vi "standupRoutine.vi"() -> ()   [LabVIEW 2013]
uses:
  <vilib>/Simulation/Implementation/XNodeFramework/SimXNode/SimX.xnode
  LinearControl.vi
  <vilib>/Simulation/Implementation/Shared/SIMSCR Execution Mode.ctl
  <vilib>/Simulation/Scripting/Companion Diagram/SimConfigNode/_simSolvers.ctl
  <vilib>/Simulation/Scripting/Companion Diagram/SimConfigNode/SimParams.ctl
  <vilib>/Simulation/Scripting/Companion Diagram/SimConfigNode/SimDog.xnode
panel:
  out "Dynamic Data Type":dynamicdata(graph)
  in  "SP_theta_e":dbl step=0.0001 format="%_6f"
  out "theta":dbl
  out "pos":dbl format="%.2f"
  out "Controller?":bool
  in  "state feedbak gain":dbl[](array[numeric])=[0.0, 0.0, 400.0, 0.0] step=1e-05 format="%_6f"
  in  "setpoint":dbl format="%_6g"
  in  "stop_swing":bool
  in  "stop_controller":bool
  in  "reset_theta":bool
  in  "reset_pos":bool
  in  "Start":bool
  in  "enable_swing":bool
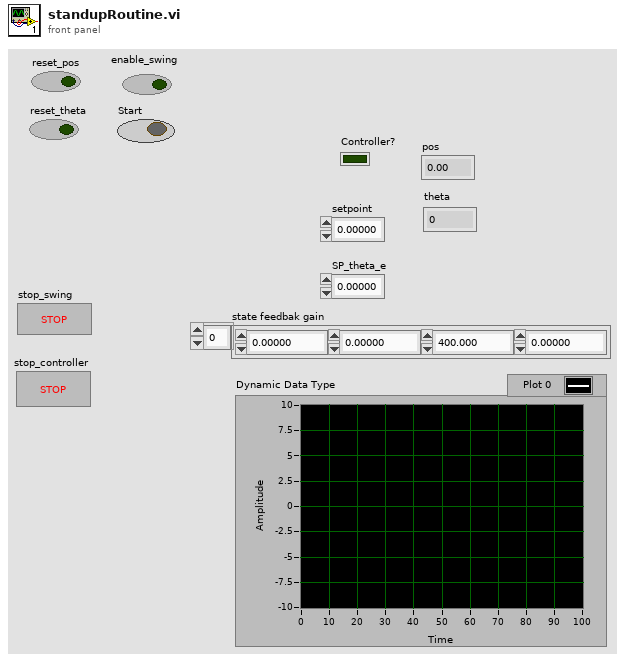
[diagram p1: front panel]
types:
  T1 = enum16{"Simulate to Completion", "Single Time-Step Simulation (Fixed Step Only)"}
  T2 = typedef "SimParams.ctl" = cluster{"Initial Time (s)":dbl, "Final Time (s)":dbl, "Step Size (s)":dbl, "ODE Solver":T3, "Minimum Step Size (s)":dbl, "Maximum Step Size (s)":dbl, "Relative Tolerance":dbl, "Absolute Tolerance":dbl, "Software Timing":bool, "Initial Step Size (s)":dbl, "Automatic Fixed Step Size?":bool, "Automatic Discrete Step Size?":bool, "Discrete Step Size (s)":dbl, "Calculate using Time Step":bool, "Solver Wired?":bool, "Prev.Frm.Expected End":u64, "Prev.Frm.Actual End":u64, "Prev.Frm.Finished Late?":bool, "Prev.Iter.Expected End":u64, "Prev.Iter.Actual End":u64, "Prev.Iter.Finished Late?":bool, "Expected Iteration Start":u64, "Actual Iteration Start":u64, "Expected Frame Start":u64, "Actual Frame Start":u64, "Source Name":string, "Name":string, "Period":i64, "Deadline":i64, "Offset":i64, "Start":i64, "Priority":i32, "Timeout":i32, "Processor":i32, "Mode":enum32{"No Change", "Process missed periods, maintain original phase", "Discard missed periods, maintain original phase", "Process missed periods, ignore original phase", "Discard missed periods, ignore original phase"}, "Wakeup reason":enum32{"Normal", "Aborted", "Asynchronous wakeup", "Timing source error", "Timed loop error", "Timeout"}, "Error":errorcluster, "Source Type":string, "Secondary Source Type":string, "Global End Time":u64, "Global Start Time":u64, "Full Solver Reset":bool, "Execution Mode":T4, "Nan/Inf Check":bool, "Custom Solver Library":string, "Solver Is Variable":bool, "custom solver name":string, "Signal Collection Decimation":u32}
  T3 = typedef "_simSolvers.ctl" = enum16{"Runge-Kutta 1 (Euler)", "Runge-Kutta 2", "Runge-Kutta 3", "Runge-Kutta 4", "Runge-Kutta 23 (variable)", "Runge-Kutta 45 (variable)", "BDF (variable)", "Adams-Moulton (variable)", "Rosenbrock (variable)", "Discrete States Only", "SDIRK 4 (variable)", "Radau 5 (variable)", "Radau 9 (variable)", "Radau 13 (variable)", "Radau [Variable Order] (variable)", "Gear's Method (variable)", "Linearizer", "State Query", "Trim Eval", "Custom Solver"}
  T4 = typedef "SIMSCR Execution Mode.ctl" = enum16{"Simulate to Completion", "Single Time-Step Simulation (Fixed Step Only)"}
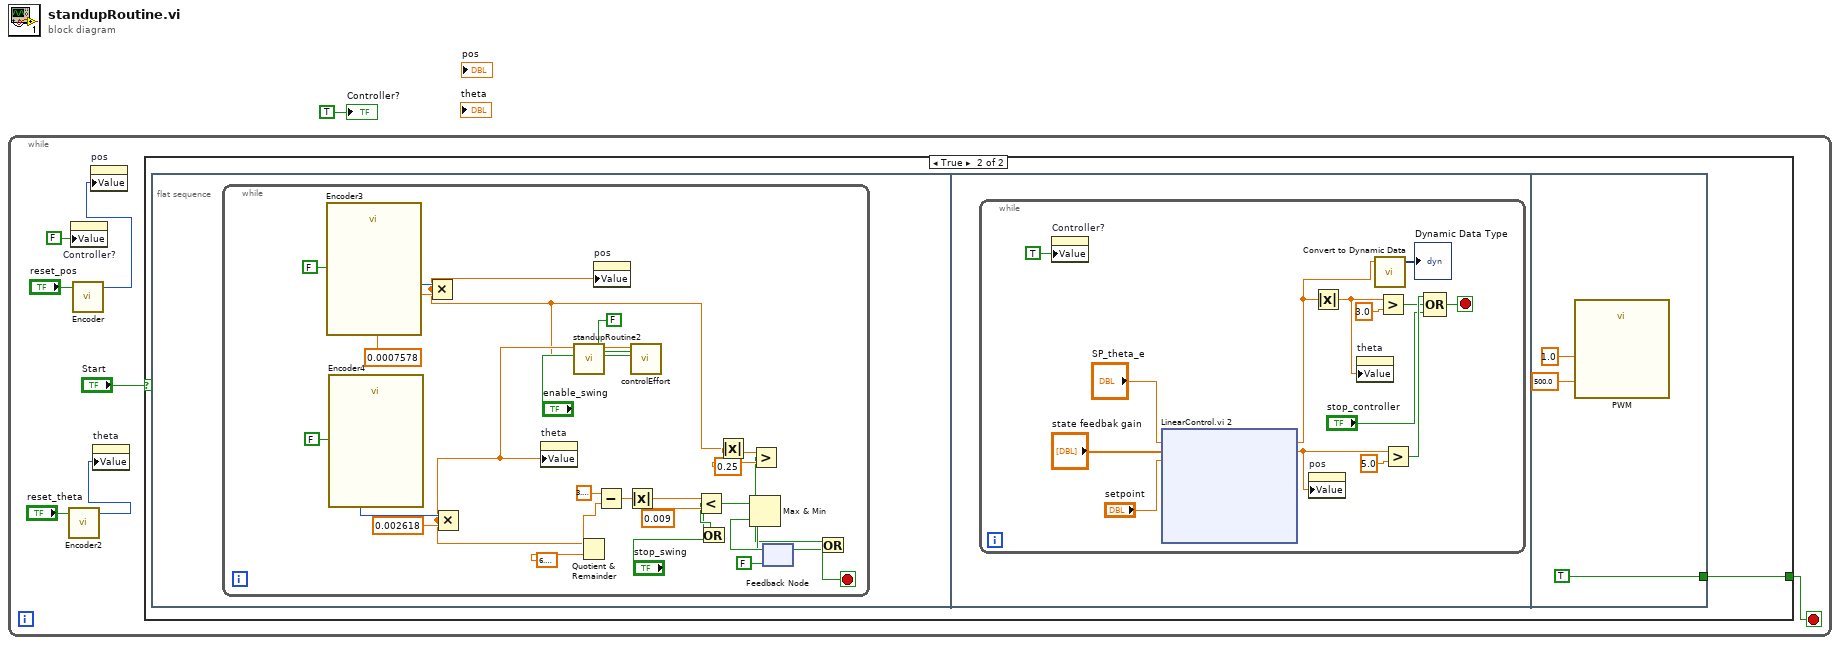
[diagram p0: block diagram]
diagram:
  n1 = while {
    stop <- w7 stop-if-true
    n2 = call "Encoder2"("Reset Counter"="reset_theta") -> ("Counter Value"=w2:i32)  [unwired: 23 in, 3 out]
    n3 = property on="Controller?" class="Bool (strict)"("Value"=FALSE ("Controller?")) -> ()  [unwired: 2 in, 2 out]
    n4 = call "Encoder"("Reset Counter"="reset_pos") -> ("Counter Value"=w3:i32)  [unwired: 23 in, 3 out]
    n5 = property on="pos" class="DigNum (strict)"("Value"=w3) -> ()  [unwired: 2 in, 2 out]
    n6 = property on="theta" class="DigNum (strict)"("Value"=w2) -> ()  [unwired: 2 in, 2 out]
    n7 = case shown="True" "Start" {
      tunnel: [_ w9] -> w7
      frame False {
      }
      frame True {
        n8 = flat-sequence {
          tunnel: [TRUE] -> w9
          frame #0 {
            n9 = while {
              stop <- w15 stop-if-true
              n10 = call "Encoder3"("Reset Counter"=FALSE) -> ("Counter Value"=w36:i32)  [unwired: 23 in, 3 out]
              n11 = call "Encoder4"("Reset Counter"=FALSE) -> ("Counter Value"=w34:i32)  [unwired: 23 in, 3 out]
              n12 = Multiply(x=w36, y=0.0007578 ("y 2")) -> (x*y=w12:dbl)
              n13 = Multiply ("Multiply 2")(x=w34, y=0.002618) -> (x*y=w16:dbl)
              n14 = property on="theta" class="DigNum (strict)"("Value"=w16) -> ()  [unwired: 2 in, 2 out]
              n15 = call "standupRoutine2.vi"("x"=w12, "theta"=w16) -> ("force"=w32:dbl)  [unwired: 9 in]
              n16 = Quotient & Remainder(x=w16, y=6.283185307179586 ("Constant")) -> (x-y*floor(x/y)=w23:dbl)  [unwired: 1 out]
              n17 = property on="pos" class="DigNum (strict)"("Value"=w12) -> ()  [unwired: 2 in, 2 out]
              n18 = Subtract(x=3.141592653589793, y=w23) -> (x-y=w24:dbl)
              n19 = Absolute Value(x=w24) -> (abs(x)=w25:dbl)
              n20 = call "controlEffort.vi"("Inverted?"=FALSE, "Enable"="enable_swing", "force"=w32) -> ()  [unwired: 9 in]
              n21 = Less?(x=w25, y=0.009) -> (x < y?=w21:bool)
              n22 = Or(x=w21, y="stop_swing") -> (x .or. y?=w19:bool)
              n23 = Absolute Value(x=w12) -> (abs(x)=w13:dbl)
              n24 = Greater?(x=w13, y=0.25) -> (0:w10:bool)
              n25 = feedback #1(FALSE) -> (w27:bool)
              n26 = Max & Min(x=w19, y=w27) -> (max(x,y)=w14:bool)  [unwired: 1 out]
              n27 = feedback-in #1(w14) -> ()
              n28 = Or(x=w10, y=w14) -> (x .or. y?=w15:bool)
            }
          }
          frame #1 {
            n29 = while {
              stop <- w44 stop-if-true
              n30 = property on="Controller?" class="Bool (strict)"("Value"=TRUE ("Controller?")) -> ()  [unwired: 2 in, 2 out]
              n31 = xnode "LinearControl.vi 2"("SP_theta_e"="SP_theta_e", "Controller Gain"="state feedbak gain", "setpoint"="setpoint") -> ("theta_e"=w38:dbl, "pos"=w40:dbl)  [unwired: 2 in, 6 out]
              n32 = property on="pos" class="DigNum (strict)"("Value"=w40) -> ()  [unwired: 2 in, 2 out]
              n33 = Absolute Value(x=w38) -> (abs(x)=w39:dbl)
              n34 = property on="theta" class="DigNum (strict)"("Value"=w39) -> ()  [unwired: 2 in, 2 out]
              n35 = call "Convert to Dynamic Data"("Double"=w38) -> ("Dynamic Data Type"=→"Dynamic Data Type":dynamicdata)  [unwired: 3 in]
              n36 = Greater?(x=w39, y=3.0) -> (0:w46:bool)
              n37 = Greater?(x=w40, y=5.0) -> (0:w47:bool)
              n38 = Compound Arithmetic op=OR(w47, w46, "stop_controller") -> (w44:bool)
            }
          }
          frame #2 {
            n39 = call "PWM"("Duty Cycle (0-1)"=1.0, "Frequency (Hz)"=500.0) -> ()  [unwired: 25 in, 1 out]
          }
        }
      }
    }
  }
  "Controller?" <- TRUE ("Boolean")
